vi "DialogManageInterfaces.vi"(8 "error in (no error)":errorcluster, 10 "ClassItemRefIn":refnum<vi>, 11 "ClassWriterNativeIn":refnum<class "ClassWriterNative.lvclass">) -> (0 "error out":errorcluster, 1 "HanldeInterfacesData":T1, 2 "Cancelled":bool, 3 "ClassWriterNativeOut":refnum<class "ClassWriterNative.lvclass">)   [LabVIEW 2020, in "ClassWriterNative.lvclass"]
uses:
  <resource>/Framework/Providers/Open_GDS/ClassProviders/Provider_LvNativeClass/ClassWriterNative_class/ClassWriterNative.lvclass
  <resource>/Framework/Providers/Open_GDS/ClassProviders/Provider_BaseClassInterface/ClassWriter_class/HandleInterfacesData.ctl
  <resource>/Framework/Providers/Open_GDS/ClassProviders/Common/InterfaceLibrary/InterfaceInfo.ctl
  <resource>/Framework/Providers/Open_GDS/ClassProviders/Common/LvClass_class/GDSLvClass_ClassMethodInfo.ctl
  <resource>/Framework/Providers/Open_GDS/ClassProviders/Provider_BaseClassInterface/ClassWriter_class/InterfacesToImplement.ctl
  <resource>/Framework/Providers/Open_GDS/ClassProviders/Common/LvClass_class/GDSLvClass_ClassInfo.ctl
  <vilib>/picture/picture.llb/imagedata.ctl
  <vilib>/Utility/miscctls.llb/LVRowAndColumnTypeDef.ctl
  <vilib>/Utility/miscctls.llb/LVRowAndColumnUnsignedTypeDef.ctl
  faae8295-b5d0-4054-ba26-443edd8c351b.vi
  a5869a5e-804e-44c9-8055-a166d2e26855.vi
  516f7541-512c-4146-8a63-54cd49fe1b68.vi
  c799aba2-3e95-4f13-9023-21e7452f1ffd.vi
  <resource>/Framework/Providers/Open_GDS/ClassProviders/Common/InterfaceLibrary/InterfaceLibrary.lvlib
  <resource>/Framework/Providers/Open_GDS/ClassProviders/Provider_BaseClassInterface/ClassWriter_class/ClassWriter.lvclass
  <resource>/Framework/Providers/_ClassSupport/Class Provider Support.lvlib
panel:
  in  "Tree":string(tree) caption="No methods selected"
  in  "_ShowContextHelp":bool
  in  "Help":bool
  in  "Cancel":bool
  in  "Save":bool
  out "ProductPicture":picture
  out "InterfaceList":i32[](listbox)
  in  "InterfaceFilter":string caption="Filter"
  out "Class":string
  # "Select Parent Interfaces (tick or untick check box)"
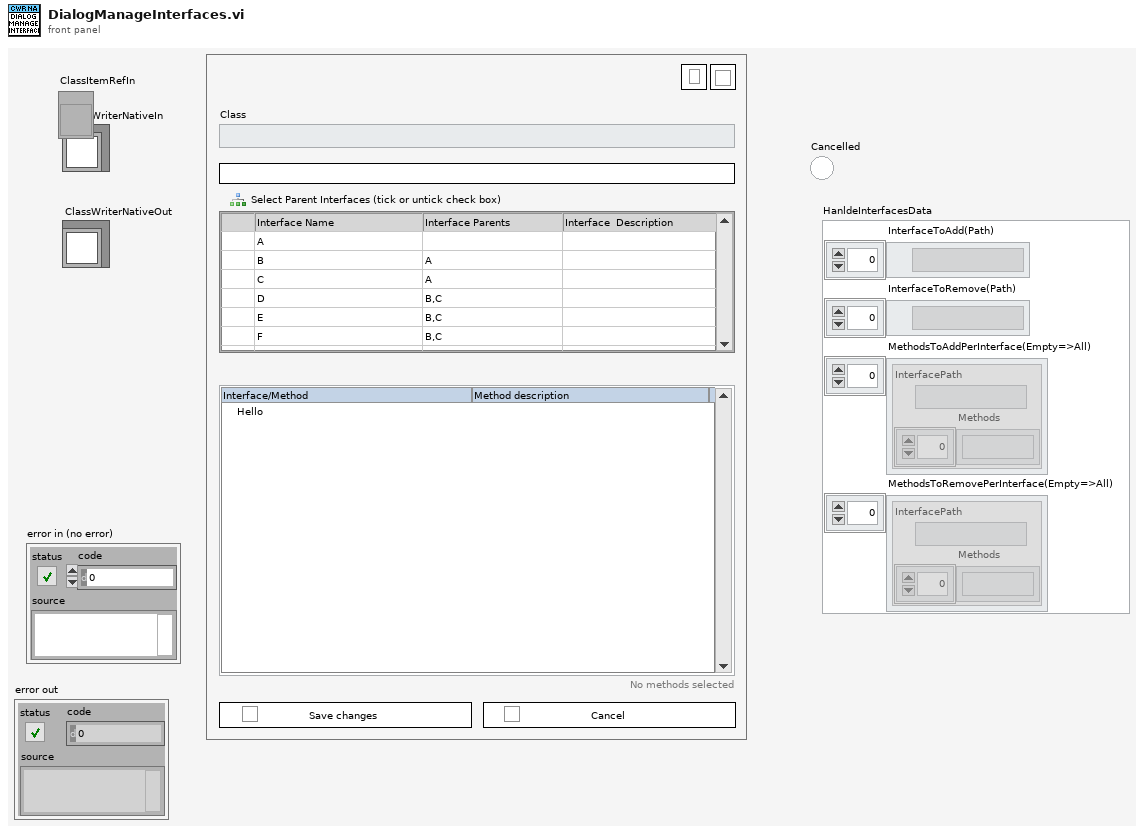
[diagram p1: front panel]
types:
  T1 = typedef "ClassWriter.lvclass/HandleInterfacesData.ctl" = cluster{"InterfaceToAdd(Path)":path[], "InterfaceToRemove(Path)":path[], "MethodsToAddPerInterface(Empty=>All)":cluster{"InterfacePath":path, "Methods":string[]}[], "MethodsToRemovePerInterface(Empty=>All)":cluster{"InterfacePath":path, "Methods":string[]}[]}
  T2 = cluster{"Font Name":string, "Size":u16, "Bold":bool, "Italic":bool, "Underline":bool, "Strikeout":bool, "Color":u32}
  T3 = typedef "InterfaceLibrary.lvlib/InterfaceInfo.ctl" = cluster{"Name(Short if no Conflicts)":string, "FullQualifierName":string, "Description":string, "Path":path, "ParentInterfaceNames(Short if no Conflitcs)":string[], "ParentInterfaceFullQualifierNames":string[], "IconPath":path, "Methods":T4[], "DynamicDispatchMethod":bool[]}
  T4 = typedef "GDSLvClass_ClassMethodInfo.ctl" = cluster{"Name":string, "Descriptions":string, "RelativePath":path, "SourceScope":enum32{"invalid scope", "public", "private", "protected", "community"}, "MustOverride":bool, "VirtualFolderLocation":string[], "DynamicDispatch":bool}
  T5 = typedef "ClassWriter.lvclass/InterfacesToImplement.ctl" = cluster{"InterfacePath":path[], "CreateMethods":bool, "MethodsPerInterface(Empty=>All)":cluster{"Methods":string[]}[]}
  T6 = typedef "GDSLvClass_ClassInfo.ctl" = cluster{"Path":path, "Name":string, "QualifiedName":string}
  T7 = cluster{"Cancel":bool, "InterfaceInfo":T3[], "IsInterface?":bool, "ParentInterfaces(path)":path[], "Interfaces(MethodsImplemented)":cluster{"Methods":string[]}[], "InterfaceIcons":path[], "VisiableInterfaceIndexes":i32[], "InterfaceSelection":enum16{"Empty", "Not", "Grey", "Blue"}[], "DisabledInterfaceIndexes":i32[], "InterfaceToAdd":T5, "InterfaceToRemove":T5, "MethodsSelectedPerInt":cluster{"Array":bool[]}[], "MethodsPerInterfaces":cluster{"Array":string[]}[], "Interfaces":string[], "StartInterfaceSelection":bool[], "Path":path, "DisabledInterafaces":i32[], "MethodsDisabledPerInt":cluster{"Array":bool[]}[], "SelectedInterfaceIndex":i32[], "ClassInheritanceHierarchy":T6[], "InterfacesParentClasesUses(path)":path[], "LvClasses":refnum<vi>[], "LvInterfaces":refnum<vi>[], "HandleInterfacesData":T1}
  T8 = typedef "imagedata.ctl" = cluster{"image type":i32, "image depth":i32, "image":u8[], "mask":u8[], "colors":u32[], "Rectangle":cluster{"left":i16, "top":i16, "right":i16, "bottom":i16}}
  T9 = typedef "LVRowAndColumnTypeDef.ctl" = cluster{"Row":i32, "Column":i32}
  T10 = typedef "LVRowAndColumnUnsignedTypeDef.ctl" = cluster{"Row":u32, "Column":u32}
  T11 = cluster{"FullQualifierInterfaceName":string, "MethodNames":string[]}[]
  T12 = cluster{"InterfacePath":path, "Methods":string[]}
  T13 = cluster{"ParentInterfaceFullQualifierNames":string[]}
  T14 = cluster{"FullQualifierName":string, "Methods":string[]}
  T15 = typedef "LVPoint32TypeDef.ctl" = cluster{"Horizontal":i32, "Vertical":i32}
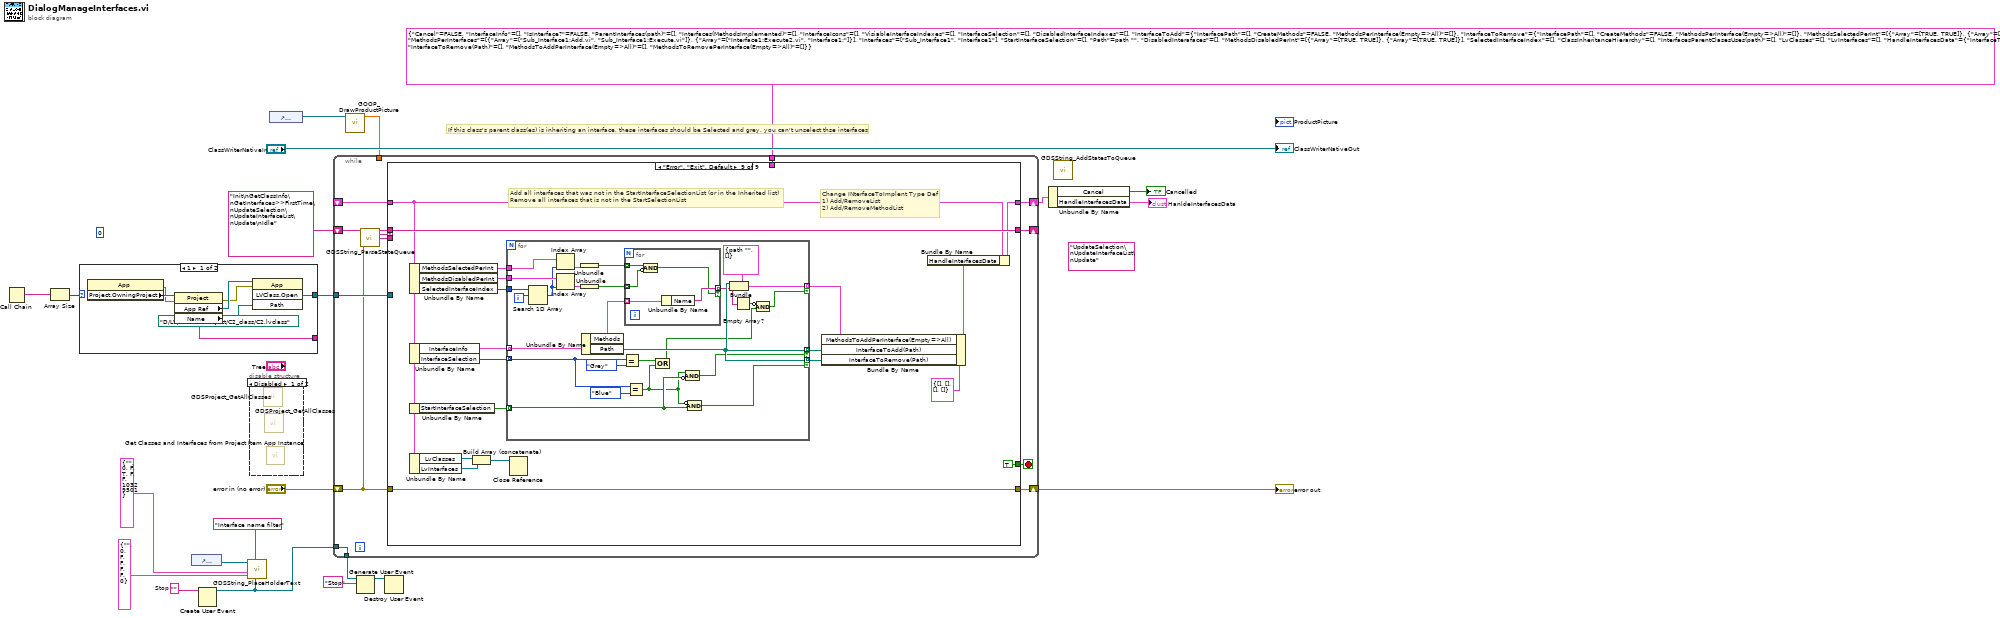
[diagram p0: block diagram]
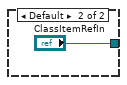
[diagram p3: hidden frame]
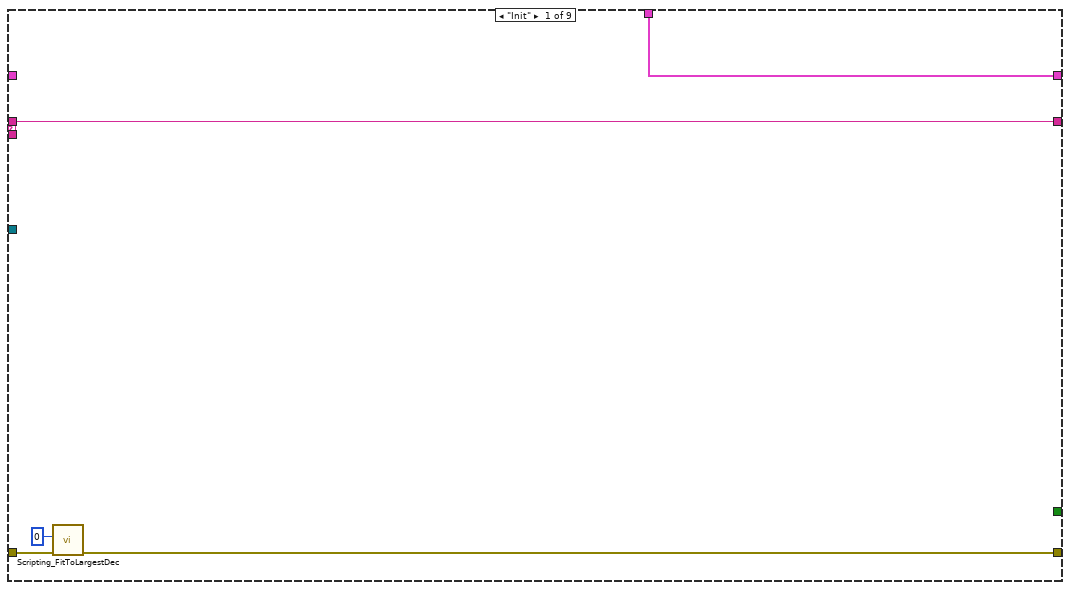
[diagram p4: hidden frame]
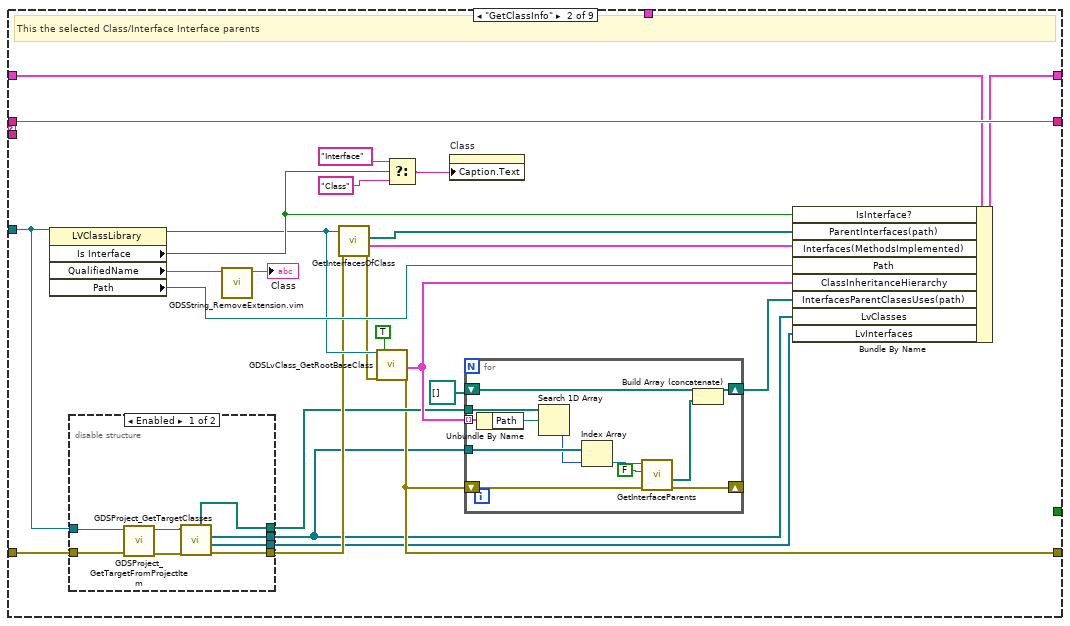
[diagram p5: hidden frame]
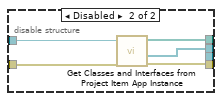
[diagram p6: hidden frame]
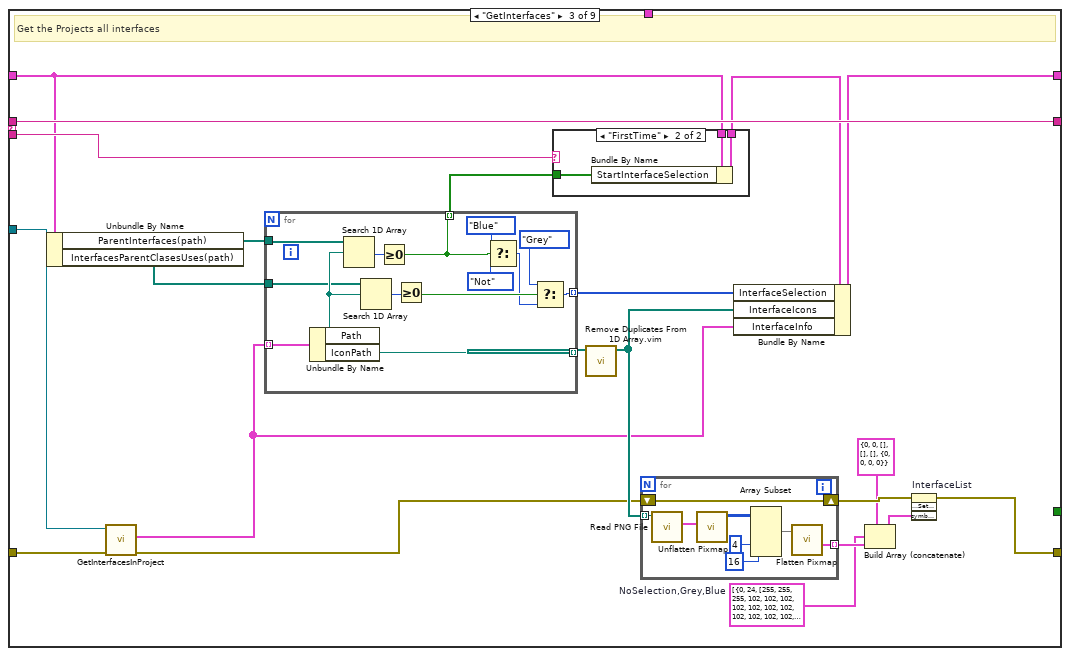
[diagram p7: hidden frame]
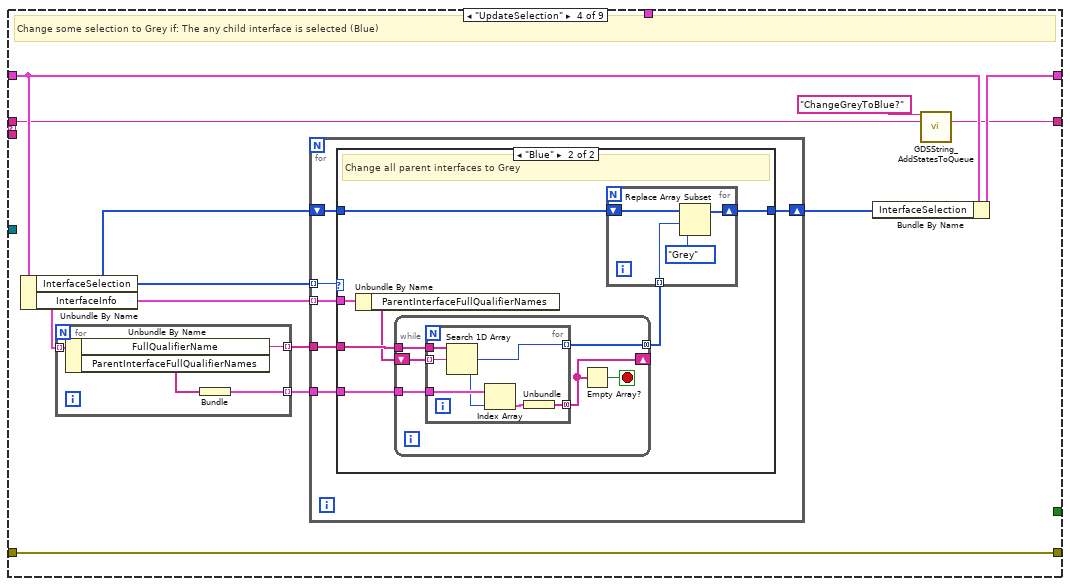
[diagram p9: hidden frame]
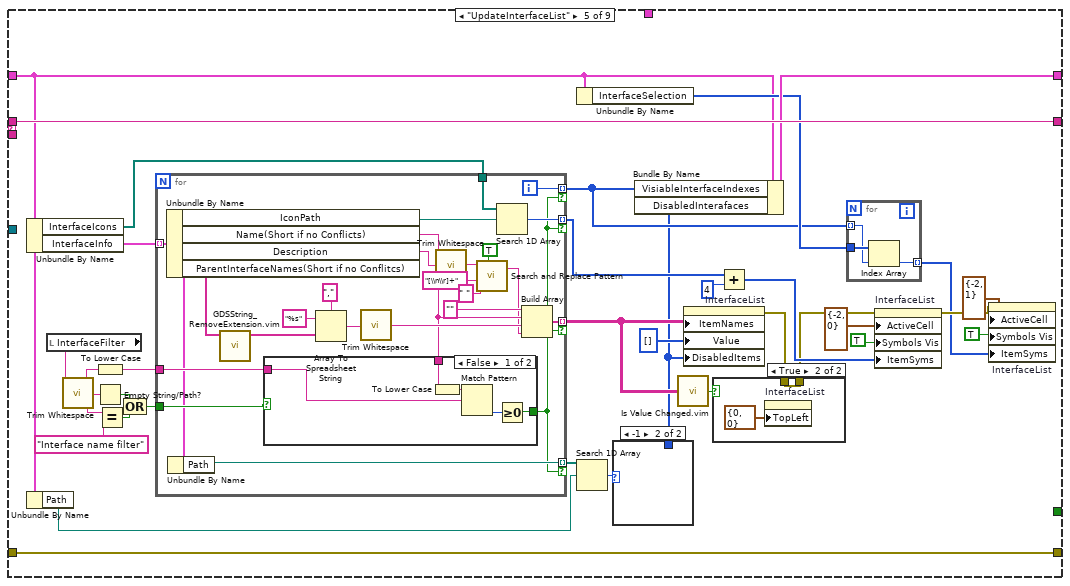
[diagram p11: hidden frame]
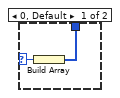
[diagram p12: hidden frame]
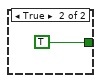
[diagram p14: hidden frame]
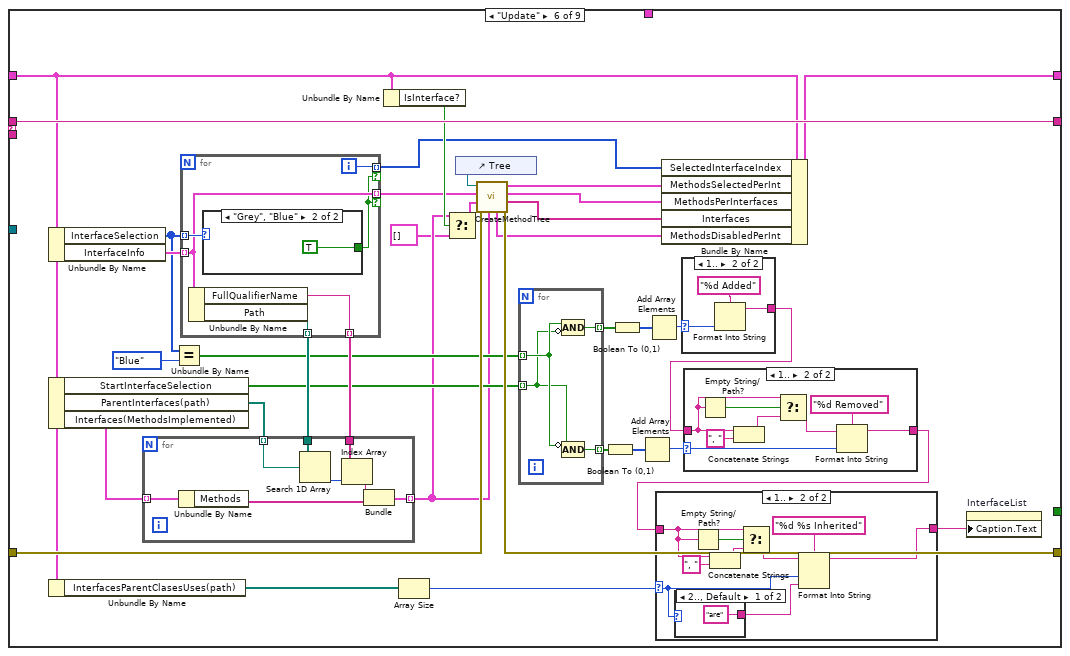
[diagram p15: hidden frame]
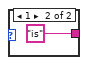
[diagram p17: hidden frame]
diagram:
  (unwired) 0
  w6 = ""  # Stop
  (unwired) "UpdateSelection\nUpdateInterfaceList\nUpdate"
  # "If this class's parent class(es) is inheriting an interface, these interfaces should be Selected and grey, you can't unselect thse interfaces"
  n1 = Call Chain() -> (call chain=w4:string[])
  n2 = Array Size(array=w4) -> (size(s)=w2:i32)
  n3 = case shown="1" w2 {
    tunnel: [w29 "ClassItemRefIn"] -> w9
    tunnel: [w23 _] -> _
    frame 1 {
      n4 = property class="App"() -> (error out=w25:errorcluster, "Project.OwningProject"=w26:refnum<vi>)  [unwired: 2 in, 1 out]
      n5 = property class="Project"(reference=w26, error in=w25) -> (error out=w24:errorcluster, "App Ref"=w27:refnum<vi>, "Name"=w23:string)  [unwired: 1 out]
      n6 = invoke class="App" method="LVClass.Open"(reference=w27, error in=w24, "Path"=path "D:/LV/RenameProject/C2_class/C2.lvclass") -> ("LVClass.Open"=w29:refnum<vi>)  [unwired: 1 in, 3 out]
    }
    frame Default {
    }
  }
  n7 = control-ref of="InterfaceFilter"() -> (w10:refnum<vi>)
  n8 = Create User Event(user event datatype=w6) -> (user event=w12:refnum<user-event>)  [unwired: 1 in, 1 out]
  n9 = call <resource>:"GDSString_PlaceHolderText.vi"("BooleanUserEventToStopPlaceHolderVI"=w12, "PlaceholderText"="Interface name filter" ("InterfaceFilter"), "PlaceholderTextFont(Grey,Italic)"=T2 {"Font Name"="", "Size"=0, "Bold"=FALSE, "Italic"=TRUE, "Underline"=FALSE, "Strikeout"=FALSE, "Color"=10329501}, "NormalTextFont(Black)"=T2 {"Font Name"="", "Size"=0, "Bold"=FALSE, "Italic"=FALSE, "Underline"=FALSE, "Strikeout"=FALSE, "Color"=0}, "PlaceholderStringRef"=w10) -> ()  [unwired: 6 in, 1 out]
  n10 = disable-structure shown="Disabled" {
    frame Disabled {
      n11 = call <resource>:"GDSProject_GetAllClasses.vi"() -> ()  [unwired: 17 in, 3 out]
      n12 = call <resource>:"GDSProject_GetAllClasses.vi"() -> ()  [unwired: 17 in, 3 out]
      n13 = call <resource>:"Get Classes and Interfaces from Project Item App Instance.vi"() -> ()  [unwired: 5 in, 7 out]
    }
    frame Enabled {
    }
  }
  n14 = control-ref of="ProductPicture"() -> (w18:refnum<vi>)
  n15 = call <resource>:"GOOP_DrawProductPicture.vi"("ProductPictureControl"=w18) -> ("Zoom Factor"=w17:sgl)  [unwired: 10 in]
  n16 = while {
    shift-right: [w42] -> w21
    shift-left: "error in (no error)" -> [w33]
    shift-right: [w39] -> _
    shift-left: "Init\nGetClassInfo\nGetInterfaces>>FirstTime\nUpdateSelection\nUpdateInterfaceList\nUpdate\nIdle" -> [w41]
    tunnel: T7 {"Cancel"=FALSE, "InterfaceInfo"=[], "IsInterface?"=FALSE, "ParentInterfaces(path)"=[], "Interfaces(MethodsImplemented)"=[], "InterfaceIcons"=[], "VisiableInterfaceIndexes"=[], "InterfaceSelection"=[], "DisabledInterfaceIndexes"=[], "InterfaceToAdd"={"InterfacePath"=[], "CreateMethods"=FALSE, "MethodsPerInterface(Empty=>All)"=[]}, "InterfaceToRemove"={"InterfacePath"=[], "CreateMethods"=FALSE, "MethodsPerInterface(Empty=>All)"=[]}, "MethodsSelectedPerInt"=[{"Array"=[TRUE, TRUE]}, {"Array"=[TRUE, TRUE]}], "MethodsPerInterfaces"=[{"Array"=["Sub_Interface1:Add.vi", "Sub_Interface1:Execute.vi"]}, {"Array"=["Interface1:Execute2.vi", "Interface1:"]}], "Interfaces"=["Sub_Interface1", "Interface1"], "StartInterfaceSelection"=[], "Path"=path "", "DisabledInterafaces"=[], "MethodsDisabledPerInt"=[{"Array"=[TRUE, TRUE]}, {"Array"=[TRUE, TRUE]}], "SelectedInterfaceIndex"=[], "ClassInheritanceHierarchy"=[], "InterfacesParentClasesUses(path)"=[], "LvClasses"=[], "LvInterfaces"=[], "HandleInterfacesData"={"InterfaceToAdd(Path)"=[], "InterfaceToRemove(Path)"=[], "MethodsToAddPerInterface(Empty=>All)"=[], "MethodsToRemovePerInterface(Empty=>All)"=[]}} -> [w36]
    shift-right: [w37] -> w8
    shift-left: _ -> [w35]
    tunnel: w9 -> [w34]
    tunnel: w17 -> [_]
    tunnel: w12 -> [w32]
    tunnel: [w32] -> w11
    stop <- w38 stop-if-true
    n17 = call <resource>:"GDSString_ParseStateQueue.vi"("State Queue"=w41, "Error In (no error)"=w33) -> ("Remaining States"=w40:string, "Current State"=w43:string, "Arguments"=w31:string)  [unwired: 9 in, 2 out]
    n18 = case shown="\"Error\", \"Exit\", Default" w43 {
      tunnel: [w45 w55 w110 w156 w223 w294 w350 w417 w483] -> w42
      tunnel: w33 -> [w46 w58 w118 w156 w223 w293 w350 w417 w483]
      tunnel: [w44 w73 w119 w147 w222 w297 w352 w412 w484] -> w39
      tunnel: w40 -> [w44 w73 w119 w148 w222 w297 _ w413 w484]
      tunnel: [_ _ _ _ _ _ _ _ TRUE] -> w38
      tunnel: [w48 w71 w116 w154 w206 w292 w351 w415 w481] -> w37
      tunnel: w36 -> [w48 _ _ _ _ _ _ _ _]
      tunnel: w35 -> [_ w72 w103 w155 w196 w266 w348 w416 w474]
      tunnel: w34 -> [_ w49 w117 _ _ _ _ _ _]
      tunnel: w31 -> [_ _ w104 _ _ _ _ _ _]
      frame "Init" {
        n19 = call <resource>:"Scripting_FitToLargestDec.vi"("error in (no error)"=w46, "border spacing (2 px)"=0) -> ("error out"=w45:errorcluster)  [unwired: 4 in, 1 out]
      }
      frame "GetClassInfo" {
        # "This the selected Class/Interface Interface parents"
        n20 = property class="LVClassLibrary"(reference=w49) -> (reference out=w61:refnum<vi>, "Is Interface"=w68:bool, "QualifiedName"=w64:string, "Path"=w62:path)  [unwired: 1 in, 1 out]
        n21 = disable-structure shown="Enabled" {
          disable-tunnel: [w81 w84] -> w59
          disable-tunnel: w58 -> [w77 w85]
          disable-tunnel: w49 -> [w75 w86]
          disable-tunnel: [w79 w83] -> w56
          disable-tunnel: [w80 w82] -> w52
          disable-tunnel: [w78 _] -> w51
          frame Enabled {
            n22 = call <resource>:"GDSProject_GetTargetFromProjectItem.vi"("error in (no error)"=w77, "ProjectItem in"=w75) -> ("error out"=w76:errorcluster, "TargetItem out"=w74:refnum<vi>)  [unwired: 8 in]
            n23 = call <resource>:"GDSProject_GetTargetClasses.vi"("error in (no error)"=w76, "TargetItem in"=w74) -> ("error out"=w81:errorcluster, "LvInterfaces"=w78:refnum<vi>[], "LvClasses"=w80:refnum<vi>[], "LvClasses(Path)"=w79:path[])  [unwired: 4 in, 2 out]
          }
          frame Disabled {
            n24 = call <resource>:"Get Classes and Interfaces from Project Item App Instance.vi"("error in"=w85, "Owning ProjectItem"=w86) -> ("error out"=w84:errorcluster, "Class Project Items"=w82:refnum<vi>[], "Class Paths"=w83:path[])  [unwired: 3 in, 4 out]
          }
        }
        n25 = call "GDSString_RemoveExtension.vim"("NameWithExtension"=w64) -> ("NameWithoutExtension"=→"Class":string)  [unwired: 10 in]
        n26 = call <resource>:"GetInterfacesOfClass.vi"("error in"=w59, "LvClassRefIn"=w61) -> ("error out"=w60:errorcluster, "Interfaces(MethodsImplemented)"=w69:cluster{"Methods":string[]}[], "Interfaces(path)"=w70:path[])  [unwired: 6 in, 1 out]
        n27 = call <resource>:"GDSLvClass_GetRootBaseClass.vi"("ViRef/Path,LvClassRef/Path"=w61, "error in (no error)"=w60, "Don'tOpenReference"=TRUE) -> ("InheritanceHierarchy"=w57:T6[], "error out"=w55:errorcluster)  [unwired: 10 in, 5 out]
        n28 = Select(t="Interface", s=w68, f="Class") -> (s? t:f=w67:string)
        n29 = property on="Class" class="Str"("Caption.Text"=w67) -> ()  [unwired: 2 in, 2 out]
        n30 = for {
          tunnel: w57 -> [w98] mode=indexing
          tunnel: w56 -> [w96]
          tunnel: w52 -> [w95]
          shift-right: [w90] -> _
          shift-left: w55 -> [w91]
          shift-right: [w92] -> w53
          shift-left: path[] [] -> [w93]
          n31 = Unbundle By Name(w98) -> ("Path"=w97:path)
          n32 = Search 1D Array(1D array=w96, element=w97) -> (index of element=w94:i32)  [unwired: 1 in]
          n33 = Index Array(array=w95, index=w94) -> (element=w89:refnum<vi>)
          n34 = call <resource>:"GetInterfaceParents.vi"("error in (no error)"=w91, "KeepRefsOpen"=FALSE, "LVClassLibrary in"=w89) -> ("error out"=w90:errorcluster, "InterfaceParents(Path)"=w87:path[])  [unwired: 5 in, 2 out]
          n35 = Build Array (concatenate)(w93, w87) -> (w92:path[])
        }
        n36 = Bundle By Name(cluster=w72, "IsInterface?"=w68, "ParentInterfaces(path)"=w70, "Interfaces(MethodsImplemented)"=w69, "Path"=w62, "ClassInheritanceHierarchy"=w57, "InterfacesParentClasesUses(path)"=w53, "LvClasses"=w52, "LvInterfaces"=w51) -> (w71:T7)
      }
      frame "GetInterfaces" {
        w105 = T8[] [{"image type"=0, "image depth"=24, "image"=[255, 255, 255, 102, 102, 102, 102, 102, 102, 102, 102, 102, 102, 102, 102, 102, 102, 102, 102, 102, 102, 102, 102, 102, 102, 102, 102, 102, 102, 102, 102, 102, 102, 102, 102, 102, 255, 255, 255, 102, 102, 102, 102, 102, 102, 102, 102, 102, 102, 102, 102, 102, 102, 102, 102, 102, 102, 102, 102, 102, 102, 102, 102, 102, 102, 102, 102, 102, 102, 102, 102, 102, 102, 102, 102, 102, 102, 102, 102, 102, 102, 102, 102, 102, 255, 255, 255, 255, 255, 255, 255, 255, 255, 255, 255, 255, 255, 255, 255, 255, 255, 255, 255, 255, 255, 255, 255, 255, 255, 255, 255, 102, 102, 102, 102, 102, 102, 102, 102, 102, 102, 102, 102, 255, 255, 255, 255, 255, 255, 255, 255, 255, 255, 255, 255, 255, 255, 255, 255, 255, 255, 255, 255, 255, 255, 255, 255, 255, 255, 255, 102, 102, 102, 102, 102, 102, 102, 102, 102, 102, 102, 102, 255, 255, 255, 255, 255, 255, 255, 255, 255, 255, 255, 255, 255, 255, 255, 255, 255, 255, 255, 255, 255, 255, 255, 255, 255, 255, 255, 102, 102, 102, 102, 102, 102, 102, 102, 102, 102, 102, 102, 255, 255, 255, 255, 255, 255, 255, 255, 255, 255, 255, 255, 255, 255, 255, 255, 255, 255, 255, 255, 255, 255, 255, 255, 255, 255, 255, 102, 102, 102, 102, 102, 102, 102, 102, 102, 102, 102, 102, 255, 255, 255, 255, 255, 255, 255, 255, 255, 255, 255, 255, 255, 255, 255, 255, 255, 255, 255, 255, 255, 255, 255, 255, 255, 255, 255, 102, 102, 102, 102, 102, 102, 102, 102, 102, 102, 102, 102, 255, 255, 255, 255, 255, 255, 255, 255, 255, 255, 255, 255, 255, 255, 255, 255, 255, 255, 255, 255, 255, 255, 255, 255, 255, 255, 255, 102, 102, 102, 102, 102, 102, 102, 102, 102, 102, 102, 102, 255, 255, 255, 255, 255, 255, 255, 255, 255, 255, 255, 255, 255, 255, 255, 255, 255, 255, 255, 255, 255, 255, 255, 255, 255, 255, 255, 102, 102, 102, 102, 102, 102, 102, 102, 102, 102, 102, 102, 255, 255, 255, 255, 255, 255, 255, 255, 255, 255, 255, 255, 255, 255, 255, 255, 255, 255, 255, 255, 255, 255, 255, 255, 255, 255, 255, 102, 102, 102, 102, 102, 102, 102, 102, 102, 102, 102, 102, 255, 255, 255, 255, 255, 255, 255, 255, 255, 255, 255, 255, 255, 255, 255, 255, 255, 255, 255, 255, 255, 255, 255, 255, 255, 255, 255, 102, 102, 102, 102, 102, 102, 102, 102, 102, 102, 102, 102, 102, 102, 102, 102, 102, 102, 102, 102, 102, 102, 102, 102, 102, 102, 102, 102, 102, 102, 102, 102, 102, 102, 102, 102, 102, 102, 102, 102, 102, 102, 102, 102, 102, 255, 255, 255, 102, 102, 102, 102, 102, 102, 102, 102, 102, 102, 102, 102, 102, 102, 102, 102, 102, 102, 102, 102, 102, 102, 102, 102, 102, 102, 102, 102, 102, 102, 102, 102, 102, 255, 255, 255], "mask"=[255, 248, 255, 248, 255, 248, 255, 248, 255, 248, 255, 248, 255, 248, 255, 248, 255, 248, 255, 248, 255, 248, 255, 248, 255, 248], "colors"=[], "Rectangle"={"left"=0, "top"=0, "right"=13, "bottom"=13}}, {"image type"=0, "image depth"=24, "image"=[255, 255, 255, 143, 143, 143, 143, 143, 143, 143, 143, 143, 143, 143, 143, 143, 143, 143, 143, 143, 143, 143, 143, 143, 143, 143, 143, 143, 143, 143, 143, 143, 143, 143, 143, 143, 255, 255, 255, 143, 143, 143, 143, 143, 143, 143, 143, 143, 143, 143, 143, 143, 143, 143, 143, 143, 143, 143, 143, 143, 143, 143, 143, 143, 143, 143, 143, 143, 143, 143, 143, 143, 170, 170, 170, 143, 143, 143, 143, 143, 143, 143, 143, 143, 143, 143, 143, 143, 143, 143, 143, 143, 143, 143, 143, 143, 143, 143, 143, 143, 143, 143, 143, 143, 143, 143, 143, 143, 170, 170, 170, 211, 211, 211, 143, 143, 143, 143, 143, 143, 143, 143, 143, 143, 143, 143, 143, 143, 143, 143, 143, 143, 143, 143, 143, 143, 143, 143, 143, 143, 143, 143, 143, 143, 170, 170, 170, 232, 232, 232, 255, 255, 255, 143, 143, 143, 143, 143, 143, 143, 143, 143, 143, 143, 143, 143, 143, 143, 143, 143, 143, 143, 143, 143, 143, 143, 143, 143, 143, 143, 170, 170, 170, 232, 232, 232, 255, 255, 255, 211, 211, 211, 143, 143, 143, 143, 143, 143, 143, 143, 143, 158, 158, 158, 143, 143, 143, 143, 143, 143, 143, 143, 143, 143, 143, 143, 170, 170, 170, 232, 232, 232, 255, 255, 255, 211, 211, 211, 143, 143, 143, 143, 143, 143, 143, 143, 143, 211, 211, 211, 218, 218, 218, 158, 158, 158, 143, 143, 143, 143, 143, 143, 170, 170, 170, 232, 232, 232, 255, 255, 255, 211, 211, 211, 154, 154, 154, 143, 143, 143, 143, 143, 143, 143, 143, 143, 226, 226, 226, 255, 255, 255, 218, 218, 218, 158, 158, 158, 170, 170, 170, 232, 232, 232, 255, 255, 255, 211, 211, 211, 154, 154, 154, 143, 143, 143, 143, 143, 143, 143, 143, 143, 143, 143, 143, 165, 165, 165, 226, 226, 226, 255, 255, 255, 218, 218, 218, 232, 232, 232, 255, 255, 255, 211, 211, 211, 154, 154, 154, 143, 143, 143, 143, 143, 143, 143, 143, 143, 143, 143, 143, 143, 143, 143, 143, 143, 143, 165, 165, 165, 226, 226, 226, 255, 255, 255, 255, 255, 255, 211, 211, 211, 154, 154, 154, 143, 143, 143, 143, 143, 143, 143, 143, 143, 143, 143, 143, 143, 143, 143, 143, 143, 143, 143, 143, 143, 143, 143, 143, 165, 165, 165, 226, 226, 226, 211, 211, 211, 154, 154, 154, 143, 143, 143, 143, 143, 143, 143, 143, 143, 143, 143, 143, 143, 143, 143, 143, 143, 143, 143, 143, 143, 143, 143, 143, 143, 143, 143, 143, 143, 143, 165, 165, 165, 154, 154, 154, 143, 143, 143, 143, 143, 143, 143, 143, 143, 143, 143, 143, 143, 143, 143, 143, 143, 143, 143, 143, 143, 255, 255, 255, 143, 143, 143, 143, 143, 143, 143, 143, 143, 143, 143, 143, 143, 143, 143, 143, 143, 143, 143, 143, 143, 143, 143, 143, 143, 143, 143, 143, 143, 143, 143, 143, 143, 255, 255, 255], "mask"=[255, 248, 255, 248, 255, 248, 255, 248, 255, 248, 255, 248, 255, 248, 255, 248, 255, 248, 255, 248, 255, 248, 255, 248, 255, 248], "colors"=[], "Rectangle"={"left"=0, "top"=0, "right"=13, "bottom"=13}}, {"image type"=0, "image depth"=24, "image"=[255, 255, 255, 33, 150, 243, 33, 150, 243, 33, 150, 243, 33, 150, 243, 33, 150, 243, 33, 150, 243, 33, 150, 243, 33, 150, 243, 33, 150, 243, 33, 150, 243, 33, 150, 243, 255, 255, 255, 33, 150, 243, 33, 150, 243, 33, 150, 243, 33, 150, 243, 33, 150, 243, 33, 150, 243, 33, 150, 243, 33, 150, 243, 33, 150, 243, 33, 150, 243, 33, 150, 243, 93, 178, 246, 33, 150, 243, 33, 150, 243, 33, 150, 243, 33, 150, 243, 33, 150, 243, 33, 150, 243, 33, 150, 243, 33, 150, 243, 33, 150, 243, 33, 150, 243, 33, 150, 243, 93, 178, 246, 174, 217, 251, 33, 150, 243, 33, 150, 243, 33, 150, 243, 33, 150, 243, 33, 150, 243, 33, 150, 243, 33, 150, 243, 33, 150, 243, 33, 150, 243, 33, 150, 243, 93, 178, 246, 214, 236, 253, 255, 255, 255, 33, 150, 243, 33, 150, 243, 33, 150, 243, 33, 150, 243, 33, 150, 243, 33, 150, 243, 33, 150, 243, 33, 150, 243, 33, 150, 243, 93, 178, 246, 214, 236, 253, 255, 255, 255, 174, 217, 251, 33, 150, 243, 33, 150, 243, 33, 150, 243, 67, 166, 245, 33, 150, 243, 33, 150, 243, 33, 150, 243, 33, 150, 243, 93, 178, 246, 214, 236, 253, 255, 255, 255, 174, 217, 251, 33, 150, 243, 33, 150, 243, 33, 150, 243, 174, 217, 251, 187, 223, 251, 67, 166, 245, 33, 150, 243, 33, 150, 243, 93, 178, 246, 214, 236, 253, 255, 255, 255, 174, 217, 251, 58, 162, 244, 33, 150, 243, 33, 150, 243, 33, 150, 243, 203, 230, 252, 255, 255, 255, 187, 223, 251, 67, 166, 245, 93, 178, 246, 214, 236, 253, 255, 255, 255, 174, 217, 251, 58, 162, 244, 33, 150, 243, 33, 150, 243, 33, 150, 243, 33, 150, 243, 82, 173, 246, 203, 230, 252, 255, 255, 255, 187, 223, 251, 214, 236, 253, 255, 255, 255, 174, 217, 251, 58, 162, 244, 33, 150, 243, 33, 150, 243, 33, 150, 243, 33, 150, 243, 33, 150, 243, 33, 150, 243, 82, 173, 246, 203, 230, 252, 255, 255, 255, 255, 255, 255, 174, 217, 251, 58, 162, 244, 33, 150, 243, 33, 150, 243, 33, 150, 243, 33, 150, 243, 33, 150, 243, 33, 150, 243, 33, 150, 243, 33, 150, 243, 82, 173, 246, 203, 230, 252, 174, 217, 251, 58, 162, 244, 33, 150, 243, 33, 150, 243, 33, 150, 243, 33, 150, 243, 33, 150, 243, 33, 150, 243, 33, 150, 243, 33, 150, 243, 33, 150, 243, 33, 150, 243, 82, 173, 246, 58, 162, 244, 33, 150, 243, 33, 150, 243, 33, 150, 243, 33, 150, 243, 33, 150, 243, 33, 150, 243, 33, 150, 243, 255, 255, 255, 33, 150, 243, 33, 150, 243, 33, 150, 243, 33, 150, 243, 33, 150, 243, 33, 150, 243, 33, 150, 243, 33, 150, 243, 33, 150, 243, 33, 150, 243, 33, 150, 243, 255, 255, 255], "mask"=[255, 248, 255, 248, 255, 248, 255, 248, 255, 248, 255, 248, 255, 248, 255, 248, 255, 248, 255, 248, 255, 248, 255, 248, 255, 248], "colors"=[], "Rectangle"={"left"=0, "top"=0, "right"=13, "bottom"=13}}]  # NoSelection,Grey,Blue
        # "Get the Projects all interfaces"
        n37 = Unbundle By Name(w103) -> ("ParentInterfaces(path)"=w108:path[], "InterfacesParentClasesUses(path)"=w100:path[])
        n38 = call <resource>:"GetInterfacesInProject.vi"("error in"=w118, "Project/ProjectItem"=w117) -> ("error out"=w111:errorcluster, "InterfaceInfo"=w99:T3[])  [unwired: 8 in]
        n39 = for {
          tunnel: w99 -> [w145] mode=indexing
          tunnel: [w144] -> w113 mode=indexing
          tunnel: w108 -> [w143]
          tunnel: [w134] -> w107 mode=indexing
          tunnel: [w132] -> w101 mode=indexing
          tunnel: w100 -> [w138]
          n40 = Unbundle By Name(w145) -> ("Path"=w139:path, "IconPath"=w144:path)
          n41 = Search 1D Array(1D array=w143, element=w139) -> (index of element=w142:i32)  [unwired: 1 in]
          n42 = Search 1D Array(1D array=w138, element=w139) -> (index of element=w137:i32)  [unwired: 1 in]
          n43 = Greater Or Equal To 0?(x=w142) -> (x >= 0?=w132:bool)
          n44 = Greater Or Equal To 0?(x=w137) -> (x >= 0?=w136:bool)
          n45 = Select(t=enum16{"Empty", "Not", "Grey", "Blue"}."Blue", s=w132, f=enum16{"Empty", "Not", "Grey", "Blue"}."Not") -> (s? t:f=w135:enum16{"Empty", "Not", "Grey", "Blue"})
          n46 = Select(t=enum16{"Empty", "Not", "Grey", "Blue"}."Grey", s=w136, f=w135) -> (s? t:f=w134:enum16{"Empty", "Not", "Grey", "Blue"})
        }
        n47 = case shown="\"FirstTime\"" w104 {
          tunnel: w103 -> [w120 w123]
          tunnel: [w120 w122] -> w102
          tunnel: w101 -> [_ w121]
          frame Default {
          }
          frame "FirstTime" {
            n48 = Bundle By Name(cluster=w123, "StartInterfaceSelection"=w121) -> (w122:T7)
          }
        }
        n49 = call "Remove Duplicates From 1D Array.vim"("array"=w113) -> ("array with duplicates removed"=w112:path[])  [unwired: 10 in]
        n50 = for {
          tunnel: w112 -> [w131] mode=indexing
          shift-right: [w125] -> w114
          shift-left: w111 -> [w125]
          tunnel: [w124] -> w115 mode=indexing
          n51 = call <vilib>:"Read PNG File.vi"("path to PNG file"=w131) -> ("image data"=w130:T8)  [unwired: 8 in, 2 out]
          n52 = call <vilib>:"Unflatten Pixmap.vi"("image data"=w130) -> ("24-bit pixmap"=w129:u32[][])  [unwired: 4 in, 6 out]
          n53 = Array Subset(array=w129, index (col)=4 ("index"), length (col)=16 ("length")) -> (w126:u32[][])  [unwired: 2 in]
          n54 = call <vilib>:"Flatten Pixmap.vi"("24-bit pixmap"=w126) -> ("image data"=w124:T8)  [unwired: 10 in]
        }
        n55 = Bundle By Name(cluster=w102, "InterfaceSelection"=w107, "InterfaceIcons"=w112, "InterfaceInfo"=w99) -> (w116:T7)
        n56 = Build Array (concatenate)(T8 {"image type"=0, "image depth"=0, "image"=[], "mask"=[], "colors"=[], "Rectangle"={"left"=0, "top"=0, "right"=0, "bottom"=0}} ("image data"), w105, w115) -> (w109:T8[])
        n57 = invoke on="InterfaceList" class="MCListbox (strict)" method="Custom Item Symbols.Set Symbol Array"(error in=w114, "symbols"=w109) -> (error out=w110:errorcluster)  [unwired: 2 in, 3 out]
      }
      frame "UpdateSelection" {
        # "Change some selection to Grey if: The any child interface is selected (Blue)"
        n58 = Unbundle By Name(w155) -> ("InterfaceSelection"=w153:enum16{"Empty", "Not", "Grey", "Blue"}[], "InterfaceInfo"=w152:T3[])
        n59 = for {
          tunnel: w152 -> [w160] mode=indexing
          tunnel: [w159] -> w151 mode=indexing
          tunnel: [w157] -> w150 mode=indexing
          n60 = Unbundle By Name(w160) -> ("FullQualifierName"=w159:string, "ParentInterfaceFullQualifierNames"=w158:string[])
          n61 = Bundle("ParentInterfaceFullQualifierNames"=w158) -> (w157:T13)  [unwired: 1 in]
        }
        n62 = for {
          tunnel: w153 -> [w166] mode=indexing
          shift-right: [w161] -> w149
          shift-left: w153 -> [w162]
          tunnel: w152 -> [w165] mode=indexing
          tunnel: w151 -> [w164]
          tunnel: w150 -> [w163]
          n63 = case shown="\"Blue\"" w166 {
            tunnel: w165 -> [_ w174]
            tunnel: w164 -> [_ w173]
            tunnel: w163 -> [_ w171]
            tunnel: w162 -> [w167 w170]
            tunnel: [w167 w168] -> w161
            frame Default {
            }
            frame "Blue" {
              # "Change all parent interfaces to Grey"
              n64 = Unbundle By Name(w174) -> ("ParentInterfaceFullQualifierNames"=w172:string[])
              n65 = while {
                tunnel: w173 -> [w184]
                shift-right: [w180] -> _
                shift-left: w172 -> [w183]
                tunnel: w171 -> [w181]
                tunnel: [w179] -> w169 mode=concatenating
                stop <- w182 stop-if-true
                n66 = for {
                  tunnel: w184 -> [w190]
                  tunnel: w183 -> [w189] mode=indexing
                  tunnel: [w187] -> w179 mode=indexing
                  tunnel: w181 -> [w188]
                  tunnel: [w185] -> w180 mode=concatenating
                  n67 = Search 1D Array(1D array=w190, element=w189) -> (index of element=w187:i32)  [unwired: 1 in]
                  n68 = Index Array(array=w188, index=w187) -> (element=w186:T13)
                  n69 = Unbundle(w186) -> ("ParentInterfaceFullQualifierNames"=w185:string[])
                }
                n70 = Empty Array?(array=w180) -> (empty?=w182:bool)
              }
              n71 = for {
                shift-right: [w177] -> w168
                shift-left: w170 -> [w178]
                tunnel: w169 -> [w176] mode=indexing
                n72 = Replace Array Subset(array=w178, new element=enum16{"Empty", "Not", "Grey", "Blue"}."Grey", index=w176) -> (w177:enum16{"Empty", "Not", "Grey", "Blue"}[])
              }
            }
          }
        }
        n73 = Bundle By Name(cluster=w155, "InterfaceSelection"=w149) -> (w154:T7)
        n74 = call <resource>:"GDSString_AddStatesToQueue.vi"("State(s) in Front (\"\")"="ChangeGreyToBlue?" ("State(s) in Front (\"\")"), "State(s) in (\"\")"=w148) -> ("States Out"=w147:string)  [unwired: 13 in]
      }
      frame "UpdateInterfaceList" {
        n75 = Unbundle By Name(w196) -> ("InterfaceIcons"=w220:path[], "InterfaceInfo"=w221:T3[])
        n76 = Unbundle By Name(w196) -> ("Path"=w194:path)
        n77 = local read "InterfaceFilter"() -> (w212:string)
        n78 = call <vilib>:"Trim Whitespace.vi"("string"=w212) -> ("trimmed string"=w216:string)  [unwired: 1 in]
        n79 = To Lower Case(string=w216) -> (all lower case string=w215:string)
        n80 = Empty String/Path?(string/path=w216) -> (empty?=w219:bool)
        n81 = Equal?(x=w216, y="Interface name filter" ("InterfaceFilter")) -> (x = y?=w218:bool)
        n82 = Compound Arithmetic op=OR(w219, w218) -> (w217:bool)
        n83 = for {
          tunnel: [w251] -> w200 mode=indexing if=w238
          tunnel: w221 -> [w241] mode=indexing
          tunnel: w220 -> [w249]
          tunnel: [w248] -> w207 mode=indexing if=w238
          tunnel: w217 -> [w247]
          tunnel: w215 -> [w245]
          tunnel: [w240] -> w192 mode=indexing if=w238
          tunnel: [w239] -> w195 mode=indexing if=w238
          i -> [w240]
          n84 = Unbundle By Name(w241) -> ("IconPath"=w250:path, "Name(Short if no Conflicts)"=w246:string, "Description"=w233:string, "ParentInterfaceNames(Short if no Conflitcs)"=w243:string[])
          n85 = Unbundle By Name(w241) -> ("Path"=w239:path)
          n86 = call "GDSString_RemoveExtension.vim"("NameWithExtension"=w243) -> ("NameWithoutExtension"=w242:string[])  [unwired: 10 in]
          n87 = case shown="False" w247 {
            tunnel: [w257 TRUE] -> w238
            tunnel: w246 -> [w260 _]
            tunnel: w245 -> [w259 _]
            frame False {
              n88 = To Lower Case(string=w260) -> (all lower case string=w256:string)
              n89 = Match Pattern(string=w256, regular expression=w259) -> (offset past match=w258:i32)  [unwired: 1 in, 3 out]
              n90 = Greater Or Equal To 0?(x=w258) -> (x >= 0?=w257:bool)
            }
            frame True {
            }
          }
          n91 = Array To Spreadsheet String(delimiter (Tab)=",", array=w242, 3:"%s" ("format string")) -> (spreadsheet string=w253:string)
          n92 = call <vilib>:"Trim Whitespace.vi"("string"=w253) -> ("trimmed string"=w252:string)  [unwired: 1 in]
          n93 = call <vilib>:"Trim Whitespace.vi"("string"=w233) -> ("trimmed string"=w237:string)  [unwired: 1 in]
          n94 = call <vilib>:"Search and Replace Pattern.vi"("string"=w237, "regular expression (\"\")"="[\\n\\r]+" ("regular expression (\"\")"), "replace string (\"\")"=" " ("replace string (\"\")"), "replace all? (F)"=TRUE) -> ("result string"=w232:string)  [unwired: 1 in, 1 out]
          n95 = Search 1D Array(1D array=w249, element=w250) -> (index of element=w248:i32)  [unwired: 1 in]
          n96 = Build Array("" ("element"), w246, w252, w232) -> (w251:string[])
        }
        n97 = Unbundle By Name(w196) -> ("InterfaceSelection"=w203:enum16{"Empty", "Not", "Grey", "Blue"}[])
        n98 = Search 1D Array(1D array=w195, element=w194) -> (index of element=w193:i32)  [unwired: 1 in]
        n99 = case shown="-1" w193 {
          selector: w193 -> [w225 _]
          tunnel: [w224 _] -> w191
          frame 0, Default {
            n100 = Build Array(w225) -> (w224:i32[])
          }
          frame -1 {
          }
        }
        n101 = Bundle By Name(cluster=w196, "VisiableInterfaceIndexes"=w192, "DisabledInterafaces"=w191) -> (w206:T7)
        n102 = call "Is Value Changed.vim"("value"=w200) -> ("changed or first call?"=w197:bool)
        n103 = property on="InterfaceList" class="MCListbox (strict)"("ItemNames"=w200, "Value"=i32[] [] ("_SelectInterfaceClass"), "DisabledItems"=w191) -> (error out=w199:errorcluster)  [unwired: 2 in, 1 out]
        n104 = case shown="True" w197 {
          tunnel: [w226 w227] -> w198
          tunnel: w199 -> [w226 w227]
          frame False {
          }
          frame True {
            n105 = property on="InterfaceList" class="MCListbox (strict)"("TopLeft"=T10 {"Row"=0, "Column"=0} ("Top Left Visible Cell")) -> ()  [unwired: 2 in, 2 out]
          }
        }
        n106 = Add(x=w207, y=4) -> (x+y=w208:i32[])
        n107 = for {
          tunnel: w192 -> [w230] mode=indexing
          tunnel: w203 -> [w231]
          tunnel: [w229] -> w201 mode=indexing
          n108 = Index Array(array=w231, index=w230) -> (element=w229:enum16{"Empty", "Not", "Grey", "Blue"})
        }
        n109 = property on="InterfaceList" class="MCListbox (strict)"(error in=w198, "ActiveCell"=T9 {"Row"=-2, "Column"=0} ("Active Cell:Active Cell"), "Symbols Vis"=TRUE ("Visible Items:Symbols Visible"), "ItemSyms"=w208) -> (error out=w202:errorcluster)  [unwired: 1 in, 1 out]
        n110 = property on="InterfaceList" class="MCListbox (strict)"(error in=w202, "ActiveCell"=T9 {"Row"=-2, "Column"=1} ("Active Cell:Active Cell"), "Symbols Vis"=TRUE ("Visible Items:Symbols Visible"), "ItemSyms"=w201) -> ()  [unwired: 1 in, 2 out]
      }
      frame "Update" {
        n111 = Unbundle By Name(w266) -> ("InterfaceSelection"=w284:enum16{"Empty", "Not", "Grey", "Blue"}[], "InterfaceInfo"=w296:T3[])
        n112 = Unbundle By Name(w266) -> ("StartInterfaceSelection"=w282:bool[], "ParentInterfaces(path)"=w287:path[], "Interfaces(MethodsImplemented)"=w288:cluster{"Methods":string[]}[])
        n113 = Unbundle By Name(w266) -> ("InterfacesParentClasesUses(path)"=w265:path[])
        n114 = Equal?(x=w284, y=enum16{"Empty", "Not", "Grey", "Blue"}."Blue") -> (x = y?=w281:bool[])
        n115 = for {
          tunnel: w296 -> [w338] mode=indexing
          tunnel: w284 -> [w339] mode=indexing
          tunnel: [w338] -> w268 mode=indexing if=w334
          tunnel: [w337] -> w286 mode=indexing
          tunnel: [w336] -> w285 mode=indexing
          tunnel: [w335] -> w267 mode=indexing if=w334
          i -> [w335]
          n116 = Unbundle By Name(w338) -> ("FullQualifierName"=w336:string, "Path"=w337:path)
          n117 = case shown="\"Grey\", \"Blue\"" w339 {
            tunnel: [_ TRUE] -> w334
            frame Default {
            }
            frame "Grey", "Blue" {
            }
          }
        }
        n118 = for {
          tunnel: w288 -> [w333] mode=indexing
          tunnel: w287 -> [w332] mode=indexing
          tunnel: w286 -> [w331]
          tunnel: w285 -> [w329]
          tunnel: [w326] -> w272 mode=indexing
          n119 = Unbundle By Name(w333) -> ("Methods"=w327:string[])
          n120 = Search 1D Array(1D array=w331, element=w332) -> (index of element=w330:i32)  [unwired: 1 in]
          n121 = Index Array(array=w329, index=w330) -> (element=w328:string)
          n122 = Bundle("FullQualifierName"=w328, "Methods"=w327) -> (w326:T14)  [unwired: 1 in]
        }
        n123 = Unbundle By Name(w266) -> ("IsInterface?"=w273:bool)
        n124 = Array Size(array=w265) -> (size(s)=w264:i32)
        n125 = Select(t=w272, s=w273, f=T11 [] ("StartSelectedMethodsPerInterfaces")) -> (s? t:f=w271:T11)
        n126 = control-ref of="Tree"() -> (w295:refnum<vi>)
        n127 = call <resource>:"CreateMethodTree.vi"("DisabledMethodsNames"=w272, "error in (no error)"=w293, "StartSelectedMethodsPerInterfaces"=w271, "InterfacePath"=w268, "TreeControlRef"=w295) -> ("error out"=w294:errorcluster, "InterfacesTag"=w289:string[], "MethodsTagPerInterfaces"=w290:cluster{"Array":string[]}[], "MethodsSelectedPerInterface"=w291:cluster{"Array":bool[]}[], "MethodsDisabledPerInterface"=w269:cluster{"Array":bool[]}[])  [unwired: 2 in]
        n128 = for {
          tunnel: w282 -> [w323] mode=indexing
          tunnel: w281 -> [w324] mode=indexing
          tunnel: [w325] -> w280 mode=indexing
          tunnel: [w322] -> w275 mode=indexing
          n129 = Compound Arithmetic op=AND(w324, invert w323) -> (w322:bool)
          n130 = Compound Arithmetic op=AND(invert w324, w323) -> (w325:bool)
        }
        n131 = Boolean To (0,1)(Boolean=w280) -> (0, 1=w279:i16[])
        n132 = Boolean To (0,1)(Boolean=w275) -> (0, 1=w276:i16[])
        n133 = Add Array Elements(numeric array=w279) -> (sum=w278:i16)
        n134 = Add Array Elements(numeric array=w276) -> (sum=w277:i16)
        n135 = Bundle By Name(cluster=w266, "SelectedInterfaceIndex"=w267, "MethodsSelectedPerInt"=w291, "MethodsPerInterfaces"=w290, "Interfaces"=w289, "MethodsDisabledPerInt"=w269) -> (w292:T7)
        n136 = case shown="1.." w277 {
          selector: w277 -> [_ w320]
          tunnel: [_ w319] -> w274
          frame 0, Default {
          }
          frame 1.. {
            n137 = Format Into String(format string="%d Added", w320) -> (resulting string=w319:string)  [unwired: 2 in, 1 out]
          }
        }
        n138 = case shown="1.." w278 {
          selector: w278 -> [_ w318]
          tunnel: [w310 w316] -> w263
          tunnel: w274 -> [w310 w313]
          frame 0, Default {
          }
          frame 1.. {
            n139 = Empty String/Path?(string/path=w313) -> (empty?=w315:bool)
            n140 = Concatenate Strings(w313, ", " ("string")) -> (w311:string)
            n141 = Select(t=w313, s=w315, f=w311) -> (s? t:f=w314:string)
            n142 = Format Into String(format string="%d Removed", initial string=w314, w318) -> (resulting string=w316:string)  [unwired: 1 in, 1 out]
          }
        }
        n143 = case shown="1.." w264 {
          selector: w264 -> [_ w300]
          tunnel: w263 -> [w298 w303]
          tunnel: [w298 w301] -> w262
          frame 0, Default {
          }
          frame 1.. {
            n144 = case shown="2.., Default" w300 {
              tunnel: ["are" ("string") "is" ("string")] -> w299
              frame 2.., Default {
              }
              frame 1 {
              }
            }
            n145 = Empty String/Path?(string/path=w303) -> (empty?=w304:bool)
            n146 = Concatenate Strings(w303, ", " ("string")) -> (w306:string)
            n147 = Select(t=w303, s=w304, f=w306) -> (s? t:f=w302:string)
            n148 = Format Into String(format string="%d %s Inherited", initial string=w302, w300, w299) -> (resulting string=w301:string)  [unwired: 1 in, 1 out]
          }
        }
        n149 = property on="InterfaceList" class="MCListbox (strict)"("Caption.Text"=w262) -> ()  [unwired: 2 in, 2 out]
      }
      frame "", "Idle" {
        n150 = event shown="[1] \"Cancel\", \"Save\": Value Change" {
          selector: _ -> [_ _ _ _ _ _ _]
          dyn-events: _ -> [_ _ _ _ _ _ _]
          timeout: _ -> [_ _ _ _ _ _ _]
          tunnel: ["Exit" "Exit" w364 _ "UpdateInterfaceList\nUpdate" _ _] -> w352
          tunnel: w348 -> [w353 w359 w365 w394 w398 w399 w401]
          tunnel: [w353 w358 w366 w390 w398 w399 w401] -> w351
          event Panel Close? {
            n151 = event-data() -> ()  [unwired: 1 in, 4 out]
            n152 = event-data("Discard?"=TRUE) -> ()  [unwired: 1 in, 1 out]
          }
          event "Cancel", "Save": Value Change {
            n153 = event-data() -> ()  [unwired: 1 in, 6 out]
            n154 = Bundle By Name(cluster=w359, "Cancel"="Cancel") -> (w358:T7)
          }
          event "InterfaceList": Mouse Down {
            n155 = event-data() -> ("Coords"=w376:T15)  [unwired: 1 in]
            n156 = Unbundle By Name(w365) -> ("DisabledInterafaces"=w362:i32[], "InterfaceSelection"=w368:enum16{"Empty", "Not", "Grey", "Blue"}[], "VisiableInterfaceIndexes"=w374:i32[])
            n157 = invoke on="InterfaceList" class="MCListbox (strict)" method="Point To Row Column"("Point"=w376) -> ("CellPosition"=w375:T9, "InGlyph"=w370:bool)  [unwired: 6 in, 5 out]
            n158 = Unbundle By Name(w375) -> ("Row"=w363:i32)
            n159 = Index Array(array=w374, index=w363) -> (element=w367:i32)
            n160 = Search 1D Array(1D array=w362, element=w363) -> (index of element=w361:i32)  [unwired: 1 in]
            n161 = Index Array(array=w368, index=w367) -> (element=w373:enum16{"Empty", "Not", "Grey", "Blue"})
            n162 = Less Than 0?(x=w361) -> (x < 0?=w360:bool)
            n163 = Not Equal?(x=w373, y=enum16{"Empty", "Not", "Grey", "Blue"}."Grey") -> (x != y?=w371:bool)
            n164 = Compound Arithmetic op=AND(w371, w370, w360) -> (w369:bool)
            n165 = case shown="False" w369 {
              tunnel: w368 -> [_ w383]
              tunnel: w367 -> [_ w382]
              tunnel: w365 -> [w377 w381]
              tunnel: [w377 w379] -> w366
              tunnel: [_ "UpdateSelection\nUpdateInterfaceList\nUpdate"] -> w364
              frame False {
              }
              frame True {
                n166 = in-place {
                  w386 = enum16{"Empty", "Not", "Grey", "Blue"}."Blue" ("y")
                  n167 = in-place-array #1(w383, w382) -> (w388:enum16{"Empty", "Not", "Grey", "Blue"})
                  n168 = Equal?(x=w388, y=w386) -> (x = y?=w387:bool)
                  n169 = Select(t=enum16{"Empty", "Not", "Grey", "Blue"}."Not" ("y"), s=w387, f=w386) -> (s? t:f=w384:enum16{"Empty", "Not", "Grey", "Blue"})
                  n170 = in-place-array #1(w384) -> (w380:enum16{"Empty", "Not", "Grey", "Blue"}[])  [unwired: 1 out]
                }
                n171 = Bundle By Name(cluster=w381, "InterfaceSelection"=w380) -> (w379:T7)
              }
            }
          }
          event "Tree": Mouse Down {
            n172 = event-data() -> ("CtlRef"=w395:refnum<vi>, "Coords"=w396:T15)  [unwired: 1 in]
            n173 = Unbundle By Name(w394) -> ("MethodsSelectedPerInt"=w393:cluster{"Array":bool[]}[], "MethodsPerInterfaces"=w392:cluster{"Array":string[]}[], "Interfaces"=w391:string[])
            n174 = call <resource>:"ChangeMethodTreeSelection.vi"("TreeControl in"=w395, "Interfaces"=w391, "MethodsPerInterfaces"=w392, "MouseClickCoordinates"=w396, "SelectedMethodsIn"=w393) -> ("SelectedMethodsOut"=w389:cluster{"Array":bool[]}[])  [unwired: 6 in]
            n175 = Bundle By Name(cluster=w394, "MethodsSelectedPerInt"=w389) -> (w390:T7)
          }
          event "InterfaceFilter": Value Change {
            n176 = event-data() -> ()  [unwired: 1 in, 6 out]
          }
          event "Help": Value Change {
            n177 = event-data() -> ()  [unwired: 1 in, 6 out]
            n178 = call <resource>:"GOOP_HelpMain.vi"() -> ()  [unwired: 12 in]
          }
          event "_ShowContextHelp": Value Change {
            n179 = event-data() -> ("NewVal"=w400:bool)  [unwired: 1 in]
            n180 = Control Help Window(1:w400) -> ()  [unwired: 1 in]
          }
        }
        n181 = Unbundle By Name(w348) -> ("MethodsSelectedPerInt"=w347:cluster{"Array":bool[]}[], "MethodsDisabledPerInt"=w346:cluster{"Array":bool[]}[])
        n182 = control-ref of="Tree"() -> (w349:refnum<vi>)
        n183 = call <resource>:"SetMethodTreeCaption.vi"("MethodsDisabledPerInt"=w346, "MethodsSelectedPerInt"=w347, "TreeControl in"=w349) -> ("Methods will be created"=w345:bool)  [unwired: 8 in]
        n184 = Select(t="Save and create methods", s=w345, f="Save changes") -> (s? t:f=w344:string)
        n185 = Build Array(w344) -> (w343:string[])
        n186 = property on="Save" class="Bool"("Strings [4]"=w343) -> ()  [unwired: 2 in, 2 out]
      }
      frame "ChangeGreyToBlue?" {
        (unwired) enum16{"Empty", "Not", "Grey", "Blue"}."Grey"
        # "If grey and no child of this is selected, change to Blue"
        n187 = Unbundle By Name(w416) -> ("InterfacesParentClasesUses(path)"=w402:path[], "InterfaceSelection"=w407:enum16{"Empty", "Not", "Grey", "Blue"}[], "InterfaceInfo"=w411:T3[])
        n188 = for {
          tunnel: w411 -> [w421] mode=indexing
          tunnel: [w420] -> w410 mode=indexing
          tunnel: [w418] -> w409 mode=indexing
          n189 = Unbundle By Name(w421) -> ("FullQualifierName"=w420:string, "ParentInterfaceFullQualifierNames"=w419:string[])
          n190 = Bundle("ParentInterfaceFullQualifierNames"=w419) -> (w418:T13)  [unwired: 1 in]
        }
        n191 = for {
          tunnel: w411 -> [w430] mode=indexing
          tunnel: [w422] -> w414 mode=concatenating if=w427
          tunnel: w407 -> [w429] mode=indexing
          tunnel: w410 -> [w426]
          tunnel: w409 -> [w425]
          n192 = Unbundle By Name(w430) -> ("ParentInterfaceFullQualifierNames"=w423:string[])
          n193 = Equal?(x=w429, y=enum16{"Empty", "Not", "Grey", "Blue"}."Blue") -> (x = y?=w427:bool)
          n194 = case shown="True" w427 {
            tunnel: w423 -> [_ w434]
            tunnel: w426 -> [_ w433]
            tunnel: w425 -> [_ w432]
            tunnel: [_ w431] -> w424
            frame False {
            }
            frame True {
              n195 = while {
                shift-right: [w435] -> _
                shift-left: w434 -> [w440]
                tunnel: [w438] -> _
                tunnel: w433 -> [w437]
                tunnel: w432 -> [w436]
                tunnel: [w435] -> w431 mode=concatenating
                stop <- w439 stop-if-true
                n196 = for {
                  tunnel: w440 -> [w446] mode=indexing
                  tunnel: [w445] -> w438 mode=indexing
                  tunnel: [w441] -> w435 mode=concatenating
                  tunnel: w437 -> [w444]
                  tunnel: w436 -> [w443]
                  n197 = Search 1D Array(1D array=w444, element=w446) -> (index of element=w445:i32)  [unwired: 1 in]
                  n198 = Index Array(array=w443, index=w445) -> (element=w442:T13)
                  n199 = Unbundle(w442) -> ("ParentInterfaceFullQualifierNames"=w441:string[])
                }
                n200 = Empty Array?(array=w435) -> (empty?=w439:bool)
              }
            }
          }
          n201 = Build Array (concatenate)(w423, w424) -> (w422:string[])
        }
        n202 = for {
          tunnel: w407 -> [w451] mode=indexing
          tunnel: w411 -> [w450] mode=indexing
          tunnel: w414 -> [w449]
          tunnel: [w448] -> w408 mode=indexing
          tunnel: w402 -> [w447]
          n203 = case shown="\"Grey\"" w451 {
            selector: w451 -> [w452 _]
            tunnel: w450 -> [_ w462]
            tunnel: w449 -> [_ w461]
            tunnel: [w452 w465] -> w448
            tunnel: w447 -> [_ w458]
            frame Default {
            }
            frame "Grey" {
              # "Should we change this to Blue?"
              n204 = Unbundle By Name(w462) -> ("Path"=w457:path, "FullQualifierName"=w460:string)
              n205 = Search 1D Array(1D array=w458, element=w457) -> (index of element=w456:i32)  [unwired: 1 in]
              n206 = Greater Or Equal To 0?(x=w456) -> (x >= 0?=w455:bool)
              n207 = Search 1D Array(1D array=w461, element=w460) -> (index of element=w459:i32)  [unwired: 1 in]
              n208 = Greater Or Equal To 0?(x=w459) -> (x >= 0?=w454:bool)
              n209 = Or(x=w455, y=w454) -> (x .or. y?=w453:bool)
              n210 = Select(t=enum16{"Empty", "Not", "Grey", "Blue"}."Grey", s=w453, f=enum16{"Empty", "Not", "Grey", "Blue"}."Blue") -> (s? t:f=w465:enum16{"Empty", "Not", "Grey", "Blue"})
            }
          }
        }
        n211 = Not Equal?(x=w407, y=w408) -> (x != y?=w406:bool)
        n212 = Select(t="UpdateSelection" ("State(s) in Front (\"\")"), s=w406, f="") -> (s? t:f=w404:string)
        n213 = Bundle By Name(cluster=w416, "InterfaceSelection"=w408) -> (w415:T7)
        n214 = call <resource>:"GDSString_AddStatesToQueue.vi"("State(s) in Front (\"\")"=w404, "State(s) in (\"\")"=w413) -> ("States Out"=w412:string)  [unwired: 13 in]
      }
      frame "Error", "Exit", Default {
        # "Change INterfaceToImplent Type Def\n1) Add/RemoveList\n2) Add/RemoveMethodList"
        # "Add all interfaces that was not in the StartInterfaceSelectionList (or in the Inherited list)\nRemove all interfaces that is not in the StartSelectionList"
        n215 = Unbundle By Name(w474) -> ("MethodsSelectedPerInt"=w468:cluster{"Array":bool[]}[], "MethodsDisabledPerInt"=w476:cluster{"Array":bool[]}[], "SelectedInterfaceIndex"=w475:i32[])
        n216 = Unbundle By Name(w474) -> ("InterfaceInfo"=w477:T3[], "InterfaceSelection"=w466:enum16{"Empty", "Not", "Grey", "Blue"}[])
        n217 = Unbundle By Name(w474) -> ("StartInterfaceSelection"=w480:bool[])
        n218 = Unbundle By Name(w474) -> ("LvClasses"=w473:refnum<vi>[], "LvInterfaces"=w472:refnum<vi>[])
        n219 = Build Array (concatenate)(w473, w472) -> (w471:refnum<vi>[])
        n220 = for {
          tunnel: w480 -> [w488] mode=indexing
          tunnel: w477 -> [w510] mode=indexing
          tunnel: [w496] -> w479 mode=indexing if=w485
          tunnel: [w496] -> w478 mode=indexing if=w509
          tunnel: w476 -> [w505]
          tunnel: [w506] -> w467 mode=indexing if=w487
          tunnel: w475 -> [w503]
          tunnel: w468 -> [w501]
          tunnel: w466 -> [w489] mode=indexing
          i -> [w502]
          n221 = Search 1D Array(1D array=w503, element=w502) -> (index of element=w500:i32)  [unwired: 1 in]
          n222 = Index Array(array=w501, index=w500) -> (element=w499:cluster{"Array":bool[]})
          n223 = Index Array(array=w505, index=w500) -> (element=w504:cluster{"Array":bool[]})
          n224 = Unbundle(w499) -> ("Array"=w498:bool[])
          n225 = Unbundle(w504) -> ("Array"=w507:bool[])
          n226 = Unbundle By Name(w510) -> ("Methods"=w508:T4[], "Path"=w496:path)
          n227 = Equal?(x=w489, y=enum16{"Empty", "Not", "Grey", "Blue"}."Grey") -> (x = y?=w491:bool)
          n228 = for {
            tunnel: w508 -> [w515] mode=indexing
            tunnel: w507 -> [w512] mode=indexing
            tunnel: [w514] -> w495 mode=indexing if=w511
            tunnel: w498 -> [w513] mode=indexing
            n229 = Compound Arithmetic op=AND(w513, invert w512) -> (w511:bool)
            n230 = Unbundle By Name(w515) -> ("Name"=w514:string)
          }
          n231 = Equal?(x=w489, y=enum16{"Empty", "Not", "Grey", "Blue"}."Blue") -> (x = y?=w486:bool)
          n232 = Compound Arithmetic op=OR(w491, w486) -> (w490:bool)
          n233 = Compound Arithmetic op=AND(w486, invert w488) -> (w485:bool)
          n234 = Compound Arithmetic op=AND(invert w486, w488) -> (w509:bool)
          n235 = Bundle(cluster=T12 {"InterfacePath"=path "", "Methods"=[]} ("Methods"), "InterfacePath"=w496, "Methods"=w495) -> (w506:T12)
          n236 = Empty Array?(array=w495) -> (empty?=w494:bool)
          n237 = Compound Arithmetic op=AND(invert w494, w490) -> (w487:bool)
        }
        n238 = Close Reference(reference=w471) -> ()  [unwired: 1 in, 1 out]
        n239 = Bundle By Name(cluster=T1 {"InterfaceToAdd(Path)"=[], "InterfaceToRemove(Path)"=[], "MethodsToAddPerInterface(Empty=>All)"=[], "MethodsToRemovePerInterface(Empty=>All)"=[]} ("HanldeInterfacesData"), "MethodsToAddPerInterface(Empty=>All)"=w467, "InterfaceToAdd(Path)"=w479, "InterfaceToRemove(Path)"=w478) -> (w469:T1)
        n240 = Bundle By Name(cluster=w474, "HandleInterfacesData"=w469) -> (w481:T7)
      }
    }
  }
  "error out" <- w21
  n241 = Generate User Event(user event=w11, event data cluster="Stop" ("Stop")) -> (user event out=w16:refnum<user-event>)  [unwired: 2 in, 1 out]
  n242 = Destroy User Event(user event=w16) -> ()  [unwired: 1 in, 1 out]
  n243 = Unbundle By Name(w8) -> ("Cancel"=→"Cancelled":bool, "HandleInterfacesData"=→"HanldeInterfacesData":T1)
  n244 = call <resource>:"GDSString_AddStatesToQueue.vi"() -> ()  [unwired: 15 in, 1 out]
  "ClassWriterNativeOut" <- "ClassWriterNativeIn"
